vi "Data.vi"(8 "error in (no error)":errorcluster, 11 "Channel Buffer DBL in":refnum<class "Channel Buffer DBL.lvclass">) -> (0 "error out":errorcluster, 2 "Channel Data":T1, 3 "Channel Buffer DBL out":refnum<class "Channel Buffer DBL.lvclass">)   [LabVIEW 2020, in "VolatusHistorian.lvlib" / "Channel Buffer DBL.lvclass"]
uses:
  Channel Buffer DBL.lvclass
  Channel Buffer DBL.lvclass/Channel Buffer DBL.ctl
  Channel Data.ctl
  VolatusHistorian.lvlib
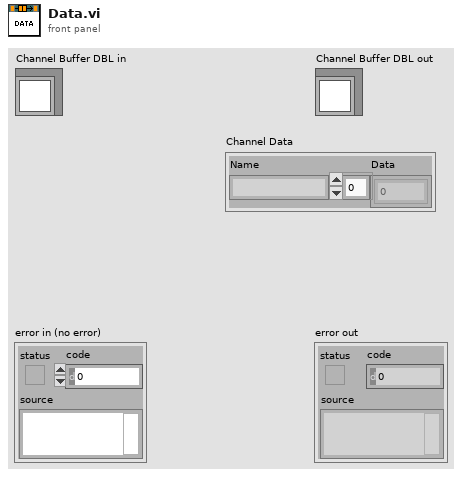
[diagram p1: front panel]
types:
  T1 = typedef "VolatusHistorian.lvlib/Channel Data.ctl" = cluster{"Name":string, "Data":dbl[]}
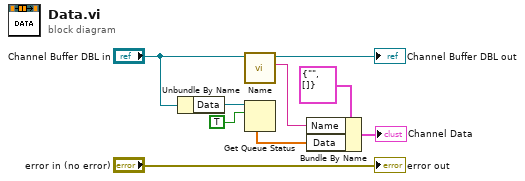
[diagram p0: block diagram]
diagram:
  n1 = Unbundle By Name("Channel Buffer DBL in") -> ("Data"=w6:refnum<queue>)
  n2 = call "Name.vi"("Channel Buffer DBL in"="Channel Buffer DBL in") -> ("Name"=w2:string, "Channel Buffer DBL out"=→"Channel Buffer DBL out":refnum<class "Channel Buffer DBL.lvclass">)  [unwired: 8 in, 1 out]
  n3 = Get Queue Status(queue=w6, return elements? (F)=TRUE) -> (elements=w1:dbl[])  [unwired: 1 in, 7 out]
  n4 = Bundle By Name(cluster=T1 {"Name"="", "Data"=[]} ("Channel Data"), "Name"=w2, "Data"=w1) -> (→"Channel Data":T1)
  "error out" <- "error in (no error)"
